vi "PQ_synchron_sample.vi"() -> ()   [LabVIEW 2019, in "libpqutility64.lvlib"]
doc: "example to evaluate c-lib functions and to show how to communicate synchronous with PostgreSQL"
uses:
  libpqutility64.lvlib
  libpqlv64/src/PQfname.vi
  libpqlv64/src/PQgetvalue.vi
  libpqlv/libpqlv.lvlib
panel:
  out "PQclientEncoding 2":i32
  out "PQsetClientEncoding":i32
  out "PQclientEncoding":i32
  out "PQoidStatus":string
  out "PQoidValue":u32
  out "PQcmdTuples":string
  out "PQcmdStatus":string
  out "PQerrorMessage":string
  out "PQresultErrorMessage":string
  in  "query":string
  out "PQresultStatus":T1(ring)
  out "PQStatus":T2(ring)
  out "PQConsumeInput":u32
  out "PQbinaryTuples":i32
  out "PQnFields":i32
  out "Tabelle":string[][](table)
  out "PQnTuples":i32
  in  "conninfo":string
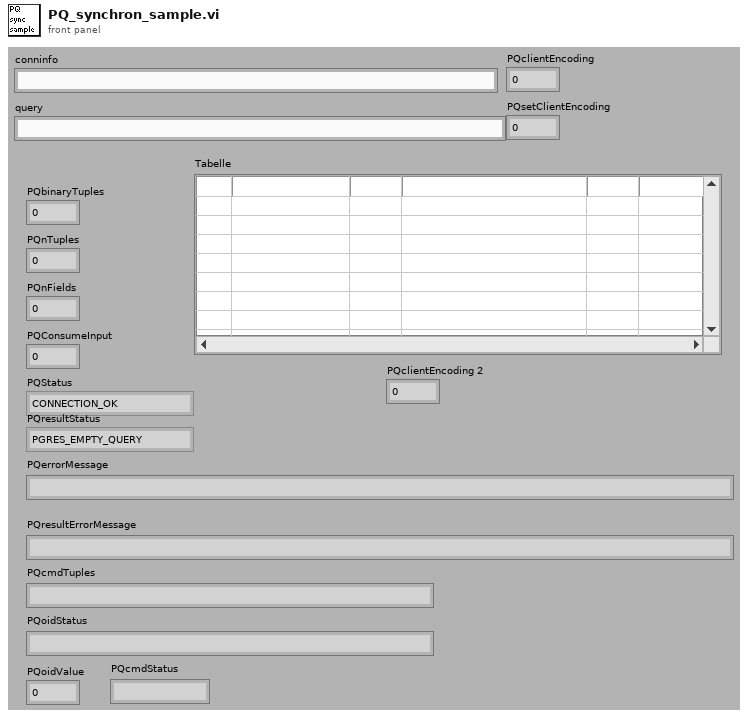
[diagram p1: front panel]
types:
  T1 = enum16{"PGRES_EMPTY_QUERY", "PGRES_COMMAND_OK", "PGRES_TUPLES_OK", "PGRES_COPY_OUT", "PGRES_COPY_IN", "PGRES_BAD_RESPONSE", "PGRES_NONFATAL_ERROR", "PGRES_FATAL_ERROR"}
  T2 = enum16{"CONNECTION_OK", "CONNECTION_BAD", "CONNECTION_STARTED", "CONNECTION_MADE", "CONNECTION_AWAITING_RESPONSE", "CONNECTION_AUTH_OK", "CONNECTION_SETENV", "CONNECTION_SSL_STARTUP", "CONNECTION_NEEDED"}
  T3 = enum32{"CONNECTION_OK", "CONNECTION_BAD", "CONNECTION_STARTED", "CONNECTION_MADE", "CONNECTION_AWAITING_RESPONSE", "CONNECTION_AUTH_OK", "CONNECTION_SETENV", "CONNECTION_SSL_STARTUP", "CONNECTION_NEEDED"}
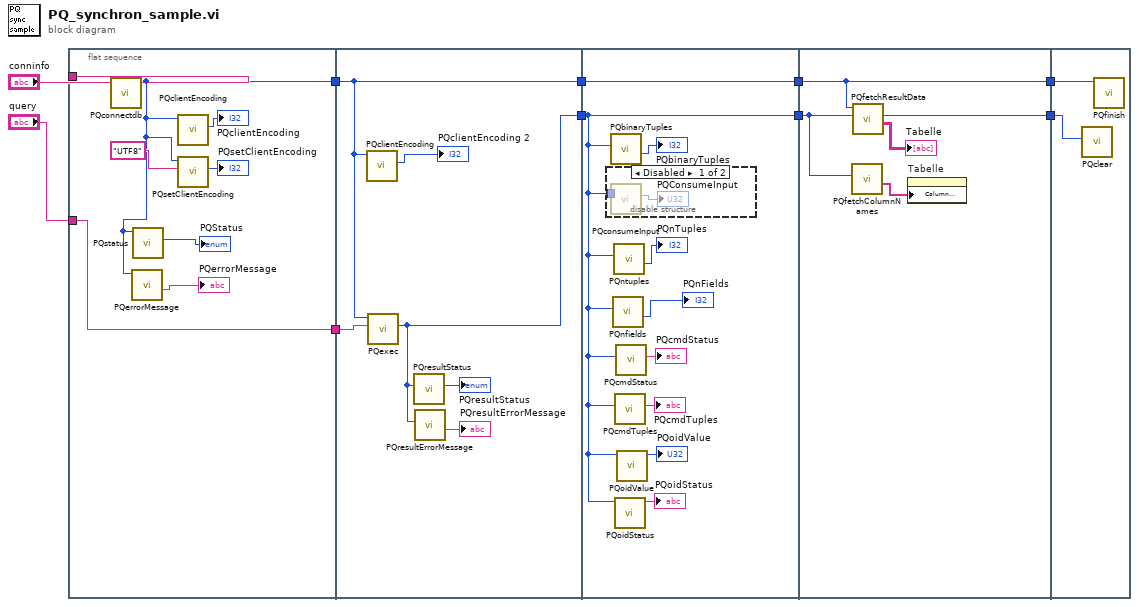
[diagram p0: block diagram]
diagram:
  n1 = flat-sequence {
    tunnel: "conninfo" -> [w18]
    tunnel: "query" -> [w14]
    tunnel: [w13] -> w3
    tunnel: [w14] -> w1
    tunnel: [w22] -> w4
    tunnel: w3 -> [w23]
    tunnel: [w23] -> w2
    tunnel: w1 -> [w24]
    tunnel: w4 -> [w29]
    tunnel: [w29] -> w7
    tunnel: w2 -> [w28]
    tunnel: [w28] -> w6
    tunnel: [w39] -> w8
    tunnel: w7 -> [w38]
    tunnel: w6 -> [w36]
    tunnel: [w36] -> w5
    tunnel: w8 -> [w42]
    tunnel: w5 -> [w41]
    frame #0 {
      n2 = call "PQconnectdb.vi"("conninfo"=w18) -> ("conn"=w13:u32)  [unwired: 9 in, 1 out]
      n3 = call "PQerrorMessage.vi"("conn"=w13) -> ("PQerrorMessage"=→"PQerrorMessage":string)  [unwired: 8 in, 2 out]
      n4 = call "PQstatus.vi"("conn"=w13) -> ("PQStatus"=→"PQStatus":T3)  [unwired: 8 in, 2 out]
      n5 = call "PQclientEncoding.vi"("conn"=w13) -> ("PQclientEncoding"=→"PQclientEncoding":i32)  [unwired: 9 in, 1 out]
      n6 = call "PQsetClientEncoding.vi"("encoding"="UTF8", "conn"=w13) -> ("PQsetClientEncoding"=→"PQsetClientEncoding":i32)  [unwired: 8 in, 1 out]
    }
    frame #1 {
      n7 = call "PQclientEncoding.vi"("conn"=w23) -> ("PQclientEncoding"=→"PQclientEncoding 2":i32)  [unwired: 9 in, 1 out]
      n8 = call "PQexec.vi"("query"=w24, "conn"=w23) -> ("PGresult"=w22:u32)  [unwired: 7 in, 2 out]
      n9 = call "PQresultStatus.vi"("res"=w22) -> ("res out"=→"PQresultStatus":u32)  [unwired: 8 in, 2 out]
      n10 = call "PQresultErrorMessage.vi"("res"=w22) -> ("PQresultErrorMessage"=→"PQresultErrorMessage":string)  [unwired: 8 in, 2 out]
    }
    frame #2 {
      n11 = disable-structure shown="Disabled" {
        disable-tunnel: w29 -> [w35 _]
        frame Disabled {
          n12 = call "PQconsumeInput.vi"("conn"=w35) -> ("PQConsumeInput"=→"PQConsumeInput":u32)  [unwired: 9 in, 1 out]
        }
        frame Enabled {
        }
      }
      n13 = call "PQbinaryTuples.vi"("res"=w29) -> ("PQbinaryTuples"=→"PQbinaryTuples":i32)  [unwired: 8 in, 2 out]
      n14 = call "PQnfields.vi"("res"=w29) -> ("PQnFields"=→"PQnFields":i32)  [unwired: 8 in, 2 out]
      n15 = call "PQntuples.vi"("res"=w29) -> ("PQnTuples"=→"PQnTuples":i32)  [unwired: 8 in, 2 out]
      n16 = call "PQcmdTuples.vi"("res"=w29) -> ("PQcmdTuples"=→"PQcmdTuples":string)  [unwired: 9 in, 1 out]
      n17 = call "PQoidStatus.vi"("res"=w29) -> ("PQoidStatus"=→"PQoidStatus":string)  [unwired: 9 in, 1 out]
      n18 = call "PQcmdStatus.vi"("res"=w29) -> ("PQcmdStatus"=→"PQcmdStatus":string)  [unwired: 9 in, 1 out]
      n19 = call "PQoidValue.vi"("res"=w29) -> ("PQoidValue"=→"PQoidValue":u32)  [unwired: 9 in, 1 out]
    }
    frame #3 {
      n20 = call "PQfetchColumnNames.vi"("res"=w38) -> ("ColumnNames"=w37:string[])  [unwired: 5 in, 3 out]
      n21 = call "PQfetchResultData.vi"("res"=w38, "conn"=w36) -> ("Data"=→"Tabelle":string[][], "res_out"=w39:u64)  [unwired: 4 in, 4 out]
      n22 = property on="Tabelle" class="Tbl (strict)"("Column Headers[]"=w37) -> ()  [unwired: 2 in, 2 out]
    }
    frame #4 {
      n23 = call "PQclear.vi"("res"=w42) -> ()  [unwired: 9 in, 2 out]
      n24 = call "PQfinish.vi"("conn"=w41) -> ()  [unwired: 10 in, 1 out]
    }
  }
